vi "Set miscData.vi"(8 "error in (no error)":errorcluster, 10 "eng_miscData":variant, 11 "AB_Build in":refnum<class "AB_Build.lvclass">) -> (0 "error out":errorcluster, 3 "AB_Build out":refnum<class "AB_Build.lvclass">)   [LabVIEW 2020, in "AB_Build.lvclass"]
uses:
  <vilib>/AppBuilder/AB_Classes/Build/AB_Build.lvclass
  <vilib>/AppBuilder/AB_Classes/Build/AB_Build.lvclass/AB_Build.ctl
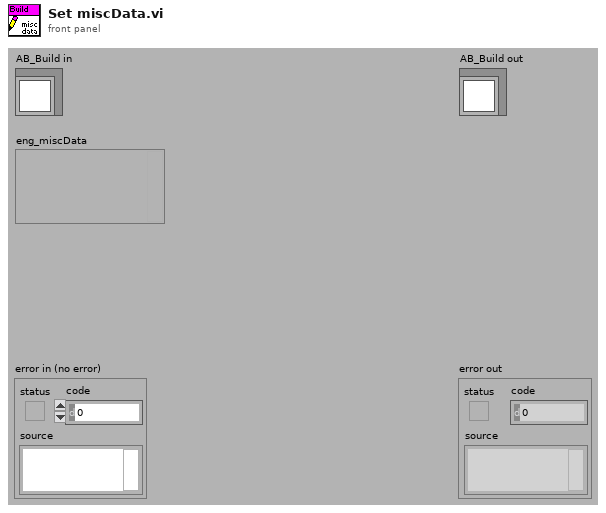
[diagram p1: front panel]
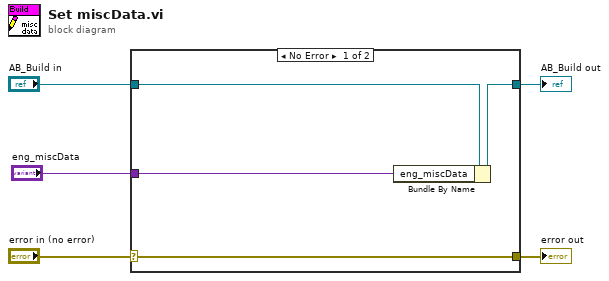
[diagram p0: block diagram]
diagram:
  n1 = case shown="No Error" "error in (no error)" {
    selector: "error in (no error)" -> [w9 w10]
    tunnel: [w9 w10] -> w4
    tunnel: [w7 w11] -> w2
    tunnel: "AB_Build in" -> [w8 w11]
    tunnel: "eng_miscData" -> [w6 _]
    frame No Error {
      n2 = Bundle By Name(cluster=w8, "eng_miscData"=w6) -> (w7:refnum<class "AB_Build.lvclass">)
    }
    frame Error {
    }
  }
  "error out" <- w4
  "AB_Build out" <- w2
